vi "Menu - String Array Del Null__SubVIs-某型振动实验台测试系统统.vi"(1 "Array":string[](array[string])) -> (0 "Out":string[](array[string]))   [LabVIEW 2011]
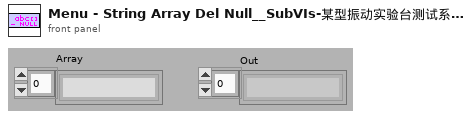
[diagram p1: front panel]
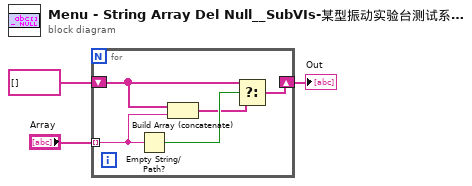
[diagram p0: block diagram]
diagram:
  n1 = for {
    tunnel: "Array" -> [w6] mode=indexing
    shift-right: [w4] -> w3
    shift-left: string[] [] -> [w7]
    n2 = Empty String/Path?(string/path=w6) -> (empty?=w8:bool)
    n3 = Build Array (concatenate)(w7, w6) -> (w5:string[])
    n4 = Select(t=w7, s=w8, f=w5) -> (s? t:f=w4:string[])
  }
  "Out" <- w3
